vi "IT-M3400 LIST_Output.vi"() -> ()   [LabVIEW 2015]
doc: "The main function of the example is to set the parameters of the list under the voltage type of the source mode and run it"
uses:
  <instrlib>/IT-M3400/IT-M3400.lvlib
panel:
  in  "Serial Configuration":T1={"Baud Rate"=9600, "Parity"=0, "Data Bits"=8, "Stop Bits"=10, "Flow Control"=0} {"Flow Control" items=["None", "XON/XOFF", "RTS/CTS", "XON/XOFF & RTS/CTS", "DTR/DSR", "XON/XOFF & DTR/DSR"]; "Stop Bits" items=["1.0"=10, "1.5"=15, "2.0"=20]; "Data Bits" items=["7"=7, "8"=8]; "Parity" items=["None", "Odd", "Even", "Mark", "Space"]; "Baud Rate" items=["300"=300, "600"=600, "1200"=1200, "2400"=2400, "4800"=4800, "9600"=9600, "19200"=19200]}
  in  "Terminate Type":u8(ring) items=["Normal", "Last"]
  in  "error in (no error)":errorcluster caption="error in(no error)"
  in  "Current limit -(A)":dbl
  in  "Current limit+(A)":dbl
  out "error out":errorcluster caption="no error"
  out "VISA resource name out":refnum<visa-resource-name>
  in  "save&recall":u8=1 min=1 max=10 step=1
  in  "Slew":dbl[](array[numeric])
  in  "Width(S)":dbl[](array[numeric])
  in  "Voltage(V)":dbl[](array[numeric])
  in  "Repeat":u32=1 min=1 step=1
  in  "Step Count":u8=1 min=1 max=100 step=1
  in  "Channel":i32(ring)=1 items=["Channel 1"=1, "Channel 2"=2, "Channel 3"=3, "Channel 4"=4, "Channel 5"=5, "Channel 6"=6, "Channel 7"=7, "Channel 8"=8, "Channel 8"=9, "Channel 10"=10, "Channel 11"=11, "Channel 12"=12, "Channel 13"=13, "Channel 14"=14, "Channel 15"=15, "Channel 16"=16]
  in  "VISA resource name":refnum<visa-resource-name>
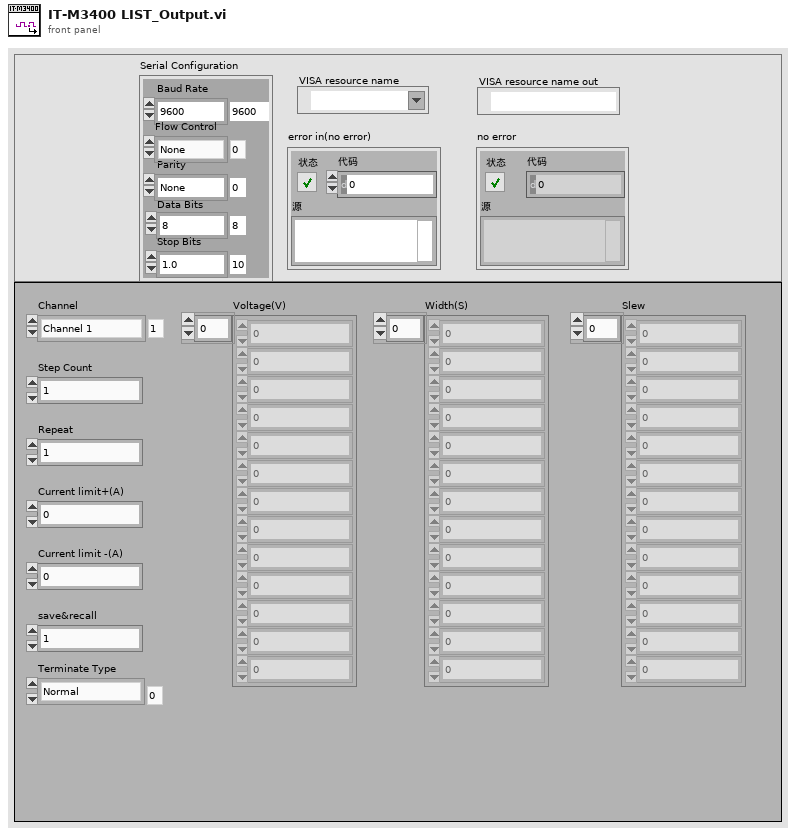
[diagram p1: front panel]
types:
  T1 = cluster{"Baud Rate":u32, "Parity":u16, "Data Bits":u16, "Stop Bits":u16, "Flow Control":u16}
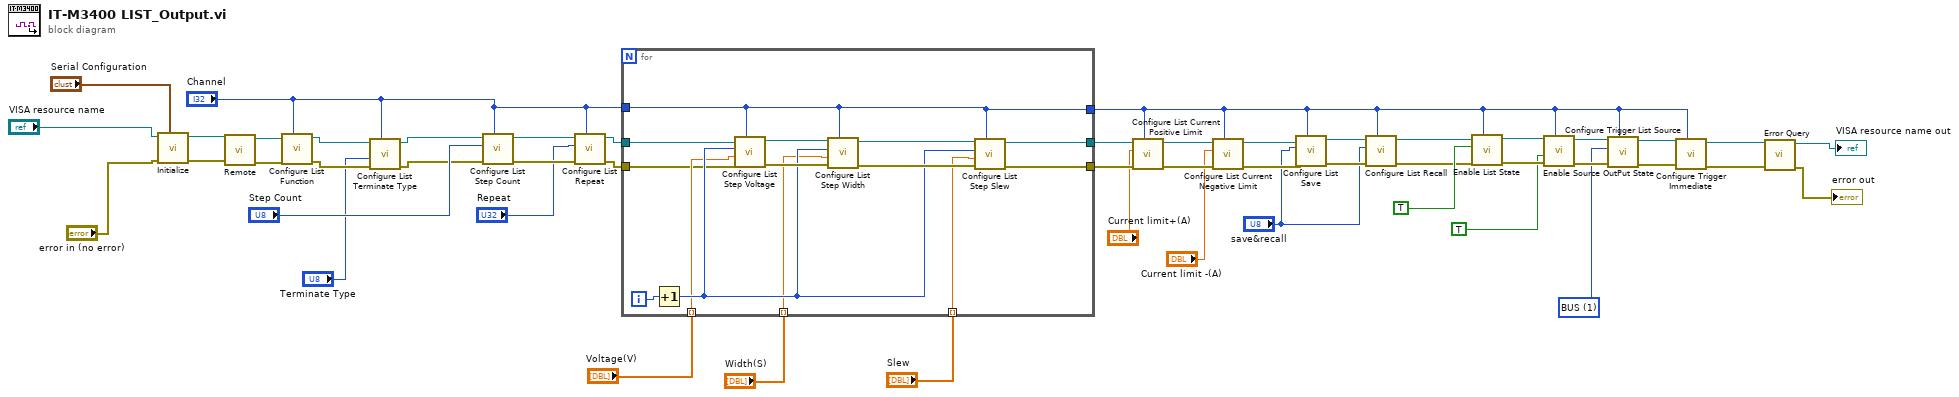
[diagram p0: block diagram]
diagram:
  w31 = u8 1 items=["KEYPad", "BUS"] ("Ponsetup Type(0:Keypad)")
  n1 = call <instrlib>:"Initialize.vi"("Serial Configuration"="Serial Configuration", "error in"="error in (no error)", "VISA resource name"="VISA resource name") -> ("error out"=w10:errorcluster, "VISA resource name out"=w11:refnum<visa-resource-name>)  [unwired: 7 in]
  n2 = call <instrlib>:"Remote.vi"("error in"=w10, "VISA resource name"=w11) -> ("error out"=w49:errorcluster, "VISA resource name out"=w48:refnum<visa-resource-name>)  [unwired: 8 in]
  n3 = call <instrlib>:"Configure List Function.vi"("Channel"="Channel", "error in"=w49, "VISA resource name"=w48) -> ("error out"=w6:errorcluster, "VISA resource name out"=w7:refnum<visa-resource-name>)  [unwired: 7 in]
  n4 = call <instrlib>:"Configure List Terminate Type.vi"("VISA resource name"=w7, "Terminate Type"="Terminate Type", "error in"=w6, "Channel"="Channel") -> ("VISA resource name out"=w5:refnum<visa-resource-name>, "error out"=w4:errorcluster)  [unwired: 5 in]
  n5 = call <instrlib>:"Configure List Step Count.vi"("Channel"="Channel", "error in"=w4, "Step Count"="Step Count", "VISA resource name"=w5) -> ("error out"=w45:errorcluster, "VISA resource name out"=w46:refnum<visa-resource-name>)  [unwired: 6 in]
  n6 = call <instrlib>:"Configure List Repeat.vi"("Channel"="Channel", "error in"=w45, "Repeat"="Repeat", "VISA resource name"=w46) -> ("error out"=w22:errorcluster, "VISA resource name out"=w23:refnum<visa-resource-name>)  [unwired: 6 in]
  n7 = for {
    tunnel: "Channel" -> [w50]
    tunnel: "Voltage(V)" -> [w57] mode=indexing
    tunnel: "Width(S)" -> [w56] mode=indexing
    tunnel: "Slew" -> [w55] mode=indexing
    tunnel: [w50] -> w15
    tunnel: w23 -> [w52]
    tunnel: [w54] -> w21
    tunnel: w22 -> [w51]
    tunnel: [w53] -> w20
    i -> [w59]
    n8 = Increment(x=w59) -> (x+1=w58:i32)
    n9 = call <instrlib>:"Configure List Step Voltage.vi"("Channel"=w50, "error in"=w51, "Voltage(V)"=w57, "Step"=w58, "VISA resource name"=w52) -> ("error out"=w62:errorcluster, "VISA resource name out"=w63:refnum<visa-resource-name>)  [unwired: 5 in]
    n10 = call <instrlib>:"Configure List Step Width.vi"("Channel"=w50, "error in"=w62, "Width(S)"=w56, "Step"=w58, "VISA resource name"=w63) -> ("error out"=w61:errorcluster, "VISA resource name out"=w60:refnum<visa-resource-name>)  [unwired: 5 in]
    n11 = call <instrlib>:"Configure List Step Slew.vi"("Channel"=w50, "error in"=w61, "Slew"=w55, "Step"=w58, "VISA resource name"=w60) -> ("error out"=w53:errorcluster, "VISA resource name out"=w54:refnum<visa-resource-name>)  [unwired: 5 in]
  }
  n12 = call <instrlib>:"Configure List Current Positive Limit.vi"("Channel"=w15, "error in"=w20, "Limit(A)"="Current limit+(A)", "VISA resource name"=w21) -> ("error out"=w18:errorcluster, "VISA resource name out"=w19:refnum<visa-resource-name>)  [unwired: 6 in]
  n13 = call <instrlib>:"Configure List Current Negative Limit.vi"("Channel"=w15, "error in"=w18, "Limit(A)"="Current limit -(A)", "VISA resource name"=w19) -> ("error out"=w16:errorcluster, "VISA resource name out"=w17:refnum<visa-resource-name>)  [unwired: 6 in]
  n14 = call <instrlib>:"Configure List Save.vi"("Channel"=w15, "error in"=w16, "File"="save&recall", "VISA resource name"=w17) -> ("error out"=w29:errorcluster, "VISA resource name out"=w30:refnum<visa-resource-name>)  [unwired: 6 in]
  n15 = call <instrlib>:"Configure List Recall.vi"("Channel"=w15, "error in"=w29, "File"="save&recall", "VISA resource name"=w30) -> ("error out"=w27:errorcluster, "VISA resource name out"=w28:refnum<visa-resource-name>)  [unwired: 6 in]
  n16 = call <instrlib>:"Enable List State.vi"("Channel"=w15, "error in"=w27, "State"=TRUE ("list状态控制"), "VISA resource name"=w28) -> ("error out"=w39:errorcluster, "VISA resource name out"=w40:refnum<visa-resource-name>)  [unwired: 6 in]
  n17 = call <instrlib>:"Enable Source OutPut State.vi"("Channel"=w15, "error in"=w39, "State"=TRUE ("ON\\OFF"), "VISA resource name"=w40) -> ("error out"=w36:errorcluster, "VISA resource name out"=w37:refnum<visa-resource-name>)  [unwired: 6 in]
  n18 = call <instrlib>:"Configure Trigger List Source.vi"("Channel"=w15, "error in"=w36, "Type"=w31, "VISA resource name"=w37) -> ("error out"=w34:errorcluster, "VISA resource name out"=w35:refnum<visa-resource-name>)  [unwired: 6 in]
  n19 = call <instrlib>:"Configure Trigger Immediate.vi"("Channel"=w15, "error in"=w34, "VISA resource name"=w35) -> ("error out"=w32:errorcluster, "VISA resource name out"=w33:refnum<visa-resource-name>)  [unwired: 7 in]
  n20 = call <instrlib>:"Error Query.vi"("error in"=w32, "VISA resource name"=w33) -> ("error out"=→"error out":errorcluster, "VISA resource name out"=→"VISA resource name out":refnum<visa-resource-name>)  [unwired: 6 in, 2 out]
